vi "AD2_SDK_Init.vi"(0 "object in":refnum<class "AD2_SDK.lvclass">, 5 "error in (no error)":errorcluster) -> (14 "object out":refnum<class "AD2_SDK.lvclass">, 19 "error out":errorcluster)   [LabVIEW 2021, in "AD2_SDK.lvclass"]
uses:
  AD2_SDK.lvclass
  AD2_MSO_SDK_class/AD2_MSO_SDK.lvclass
  AD2_WFG_SDK_class/AD2_WFG_SDK.lvclass
  AD2_DO_SDK_class/AD2_DO_SDK.lvclass
  AD2_SDK.lvclass/AD2_SDK.ctl
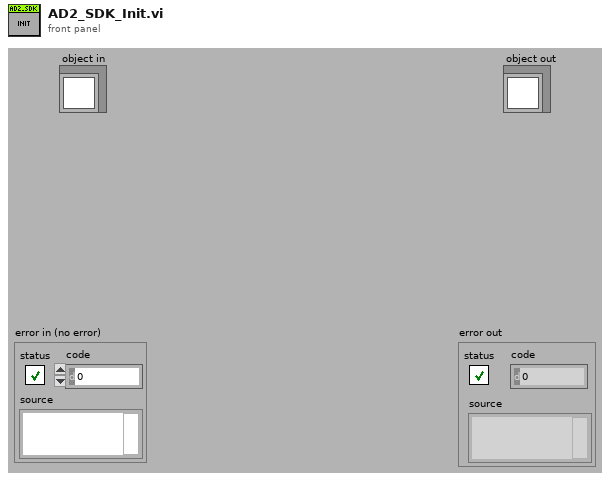
[diagram p1: front panel]
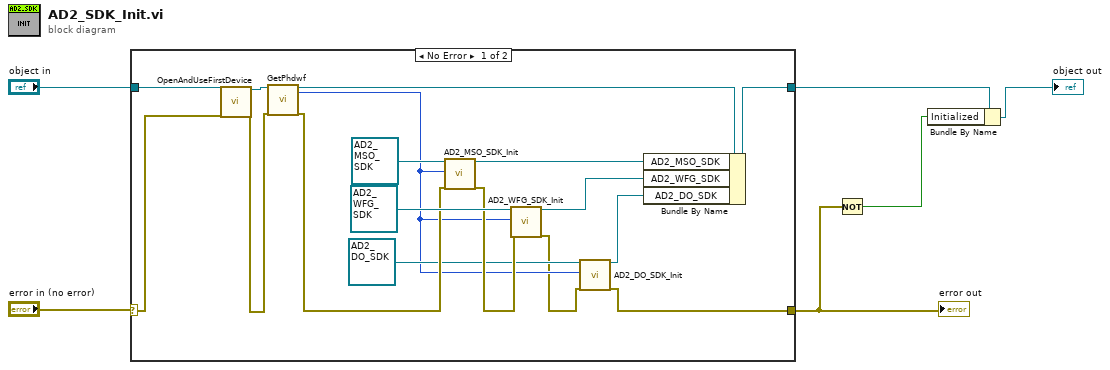
[diagram p0: block diagram]
diagram:
  n1 = case shown="No Error" "error in (no error)" {
    selector: "error in (no error)" -> [w12 w24]
    tunnel: "object in" -> [w13 w25]
    tunnel: [w23 w25] -> w4
    tunnel: [w8 w24] -> w2
    frame No Error {
      n2 = call-dynamic "OpenAndUseFirstDevice.vi"("object in"=w13, "error in (no error)"=w12) -> ("object out"=w20:refnum<class "AD2_SDK.lvclass">, "error out"=w19:errorcluster)  [unwired: 16 in]
      n3 = call-dynamic "GetPhdwf.vi"("object in"=w20, "error in (no error)"=w19) -> ("object out"=w14:refnum<class "AD2_SDK.lvclass">, "phdwf"=w10:i32, "error out"=w15:errorcluster)  [unwired: 15 in]
      n4 = call "AD2_MSO_SDK_Init.vi"("object in"=refnum<class "AD2_MSO_SDK.lvclass"> refnum ("AD2_MSO_SDK"), "phdwf"=w10, "error in (no error)"=w15) -> ("object out"=w17:refnum<class "AD2_MSO_SDK.lvclass">, "error out"=w16:errorcluster)  [unwired: 15 in]
      n5 = call "AD2_WFG_SDK_Init.vi"("object in"=refnum<class "AD2_WFG_SDK.lvclass"> refnum ("AD2_SDK"), "phdwf"=w10, "error in (no error)"=w16) -> ("object out"=w21:refnum<class "AD2_WFG_SDK.lvclass">, "error out"=w9:errorcluster)  [unwired: 15 in]
      n6 = call "AD2_DO_SDK_Init.vi"("object in"=refnum<class "AD2_DO_SDK.lvclass"> refnum ("AD2_DO_SDK"), "phdwf"=w10, "error in (no error)"=w9) -> ("object out"=w7:refnum<class "AD2_DO_SDK.lvclass">, "error out"=w8:errorcluster)  [unwired: 15 in]
      n7 = Bundle By Name(cluster=w14, "AD2_MSO_SDK"=w17, "AD2_WFG_SDK"=w21, "AD2_DO_SDK"=w7) -> (w23:refnum<class "AD2_SDK.lvclass">)
    }
    frame Error {
    }
  }
  "error out" <- w2
  n8 = Not(x=w2) -> (.not. x?=w1:bool)
  n9 = Bundle By Name(cluster=w4, "Initialized"=w1) -> (→"object out":refnum<class "AD2_SDK.lvclass">)
